vi "Set Object Count.vi"(9 "Num Cans":i32, 11 "Num Totes":i32) -> ()   [LabVIEW 2014]
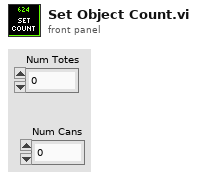
[diagram p1: front panel]
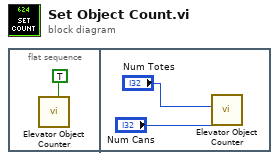
[diagram p0: block diagram]
diagram:
  n1 = flat-sequence {
    frame #0 {
      n2 = call "Elevator Object Counter.vi"("Clear Stack?"=TRUE) -> ()  [unwired: 9 in, 2 out]
    }
    frame #1 {
      n3 = call "Elevator Object Counter.vi"("Trashcan Delta"="Num Cans", "Tote Delta"="Num Totes") -> ()  [unwired: 8 in, 2 out]
    }
  }
